vi "GenerateLAB Histo.vi"(9 "Lighting":u16(ring)=5 items=["Incandescent/tungsten", "Old direct sunlight at noon", "Old daylight", "ICC profile PCS", "Mid-morning daylight", "Daylight, sRGB, Adobe-RGB", "North sky daylight", "Equal energy", "Daylight Fluorescent", "Cool fluorescent", "White Fluorescent", "Warm White Fluorescent", "Daylight Fluorescent", "Lite White Fluorescent", "Daylight fluorescent, D65 simulator", "Sylvania F40, D50 simulator", "Cool White Fluorescent", "Ultralume 50, Philips TL85", "Ultralume 40, Philips TL84", "Ultralume 30, Philips TL83"], 11 "2D Picture":picture) -> (1 "Dimensions":string, 3 "Plots":T1)   [LabVIEW 2020]
panel:
  out "b":dbl[](graph)
  out "a":dbl[](graph)
  out "L":dbl[](graph)
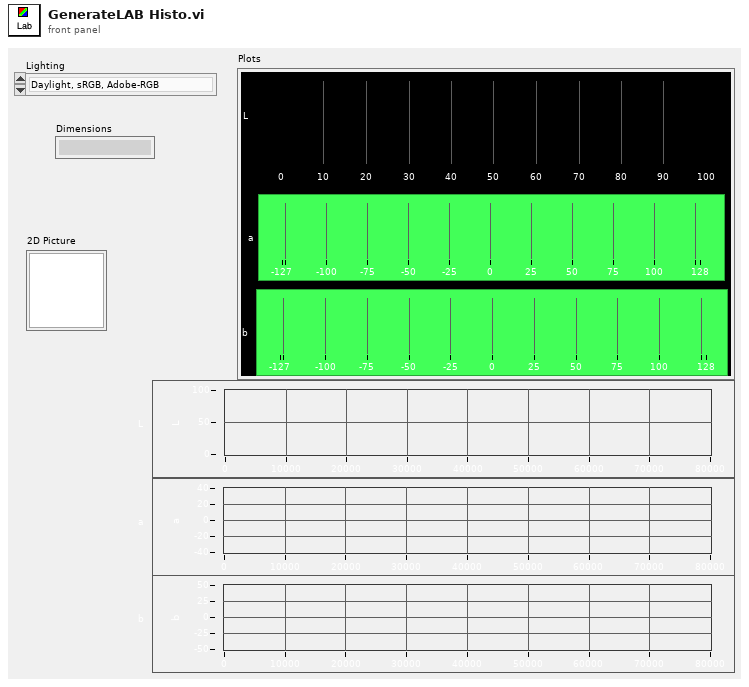
[diagram p1: front panel]
types:
  T1 = cluster{"L":dbl[], "a":cluster{i32, i32, dbl[]}, "b":cluster{i32, i32, dbl[]}}
  T2 = typedef "imagedata.ctl" = cluster{"image type":i32, "image depth":i32, "image":u8[], "mask":u8[], "colors":u32[], "Rectangle":cluster{"left":i16, "top":i16, "right":i16, "bottom":i16}}
  T3 = cluster{dbl[], cluster{i32, i32, dbl[]}, cluster{i32, i32, dbl[]}}
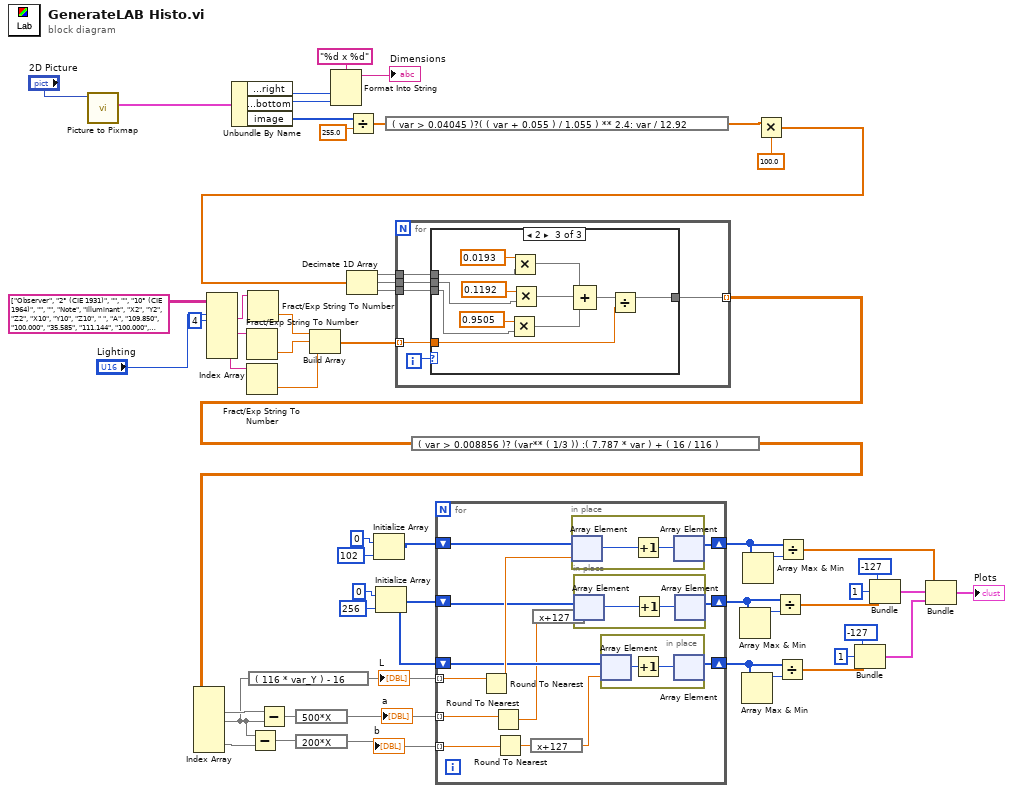
[diagram p0: block diagram]
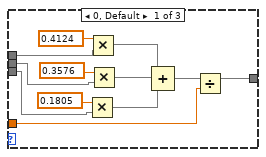
[diagram p2: hidden frame]
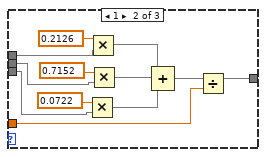
[diagram p3: hidden frame]
diagram:
  n1 = call <vilib>:"Picture to Pixmap.vi"("picture"="2D Picture") -> ("image data"=w1:T2)  [unwired: 9 in, 1 out]
  n2 = Index Array(array=string[][] [["Observer", "2° (CIE 1931)", "", "", "10° (CIE 1964)", "", "", "Note"], ["Illuminant", "X2", "Y2", "Z2", "X10", "Y10", "Z10", " "], ["A", "109.850", "100.000", "35.585", "111.144", "100.000", "35.200", "Incandescent/tungsten"], ["B", "99.0927", "100.000", "85.313", "99.178;", "100.000", "84.3493", "Old direct sunlight at noon"], ["C", "98.074", "100.000", "118.232", "97.285", "100.000", "116.145", "Old daylight"], ["D50", "96.422", "100.000", "82.521", "96.720", "100.000", "81.427", "ICC profile PCS"], ["D55", "95.682", "100.000", "92.149", "95.799", "100.000", "90.926", "Mid-morning daylight"], ["D65", "95.047", "100.000", "108.883", "94.811", "100.000", "107.304", "Daylight, sRGB, Adobe-RGB"], ["D75", "94.972", "100.000", "122.638", "94.416", "100.000", "120.641", "North sky daylight"], ["E", "100.000", "100.000", "100.000", "100.000", "100.000", "100.000", "Equal energy"], ["F1", "92.834", "100.000", "103.665", "94.791", "100.000", "103.191", "Daylight Fluorescent"], ["F2", "99.187", "100.000", "67.395", "103.280", "100.000", "69.026", "Cool fluorescent"], ["F3", "103.754", "100.000", "49.861", "108.968", "100.000", "51.965", "White Fluorescent"], ["F4", "109.147", "100.000", "38.813", "114.961", "100.000", "40.963", "Warm White Fluorescent"], ["F5", "90.872", "100.000", "98.723", "93.369", "100.000", "98.636", "Daylight Fluorescent"], ["F6", "97.309", "100.000", "60.191", "102.148", "100.000", "62.074", "Lite White Fluorescent"], ["F7", "95.044", "100.000", "108.755", "95.792", "100.000", "107.687", "Daylight fluorescent, D65 simulator"], ["F8", "96.413", "100.000", "82.333", "97.115", "100.000", "81.135", "Sylvania F40, D50 simulator"], ["F9", "100.365", "100.000", "67.868", "102.116", "100.000", "67.826", "Cool White Fluorescent"], ["F10", "96.174", "100.000", "81.712", "99.001", "100.000", "83.134", "Ultralume 50, Philips TL85"], ["F11", "100.966", "100.000", "64.370", "103.866", "100.000", "65.627", "Ultralume 40, Philips TL84"], ["F12", "108.046", "100.000", "39.228", "111.428", "100.000", "40.353", "Ultralume 30, Philips TL83"]] ("Table Control"), index (row) #1="Lighting", index (col) #1=4 ("index (col)")) -> (element #1=w14:string, element #2=w13:string, element #3=w12:string)  [unwired: 4 in]
  n3 = Unbundle By Name(w1) -> ("Rectangle.right"=w18:i16, "Rectangle.bottom"=w17:i16, "image"=w39:u8[])
  n4 = Fract/Exp String To Number(string=w13) -> (number=w8:dbl)  [unwired: 3 in, 1 out]
  n5 = Fract/Exp String To Number(string=w12) -> (number=w7:dbl)  [unwired: 3 in, 1 out]
  n6 = Fract/Exp String To Number(string=w14) -> (number=w9:dbl)  [unwired: 3 in, 1 out]
  n7 = Build Array(w9, w8, w7) -> (w6:dbl[])
  n8 = Format Into String(format string="%d x %d", w18, w17) -> (resulting string=→"Dimensions":string)  [unwired: 2 in, 1 out]
  n9 = Divide(x=w39, y=255.0) -> (x/y=w56:dbl[])
  n10 = Initialize Array(u32 0, 102 ("dimension size")) -> (w36:u32[])
  n11 = Initialize Array(u32 0, 256 ("dimension size")) -> (w43:u32[])
  n12 = expression code="( var > 0.04045 )?( ( var + 0.055 ) / 1.055 ) ** 2.4: var / 12.92"(w56) -> (w41:dbl[])
  n13 = Multiply(x=w41, y=100.0) -> (x*y=w40:dbl[])
  n14 = Decimate 1D Array(w40) -> (w55:dbl[], w54:dbl[], w53:dbl[])
  n15 = for {
    tunnel: w55 -> [w62]
    tunnel: w54 -> [w61]
    tunnel: w53 -> [w60]
    tunnel: [w59] -> w52 mode=indexing
    tunnel: w6 -> [w58] mode=indexing
    i -> [w63]
    n16 = case shown="2" w63 {
      tunnel: w62 -> [w74 w86 w98]
      tunnel: w61 -> [w73 w85 w97]
      tunnel: w60 -> [w72 w84 w96]
      tunnel: [w65 w77 w89] -> w59
      tunnel: w58 -> [w64 w76 w88]
      frame 0, Default {
        n17 = Multiply(x=0.1805, y=w72) -> (x*y=w67:dbl[])
        n18 = Multiply(x=0.4124, y=w74) -> (x*y=w68:dbl[])
        n19 = Multiply(x=0.3576, y=w73) -> (x*y=w69:dbl[])
        n20 = Compound Arithmetic op=ADD(w68, w69, w67) -> (w66:dbl[])
        n21 = Divide(x=w66, y=w64) -> (x/y=w65:dbl[])
      }
      frame 1 {
        n22 = Multiply(x=0.0722, y=w84) -> (x*y=w79:dbl[])
        n23 = Multiply(x=0.2126, y=w86) -> (x*y=w80:dbl[])
        n24 = Multiply(x=0.7152, y=w85) -> (x*y=w81:dbl[])
        n25 = Compound Arithmetic op=ADD(w80, w81, w79) -> (w78:dbl[])
        n26 = Divide(x=w78, y=w76) -> (x/y=w77:dbl[])
      }
      frame 2 {
        n27 = Multiply(x=0.9505, y=w96) -> (x*y=w91:dbl[])
        n28 = Multiply(x=0.0193, y=w98) -> (x*y=w92:dbl[])
        n29 = Multiply(x=0.1192, y=w97) -> (x*y=w93:dbl[])
        n30 = Compound Arithmetic op=ADD(w92, w93, w91) -> (w90:dbl[])
        n31 = Divide(x=w90, y=w88) -> (x/y=w89:dbl[])
      }
    }
  }
  n32 = expression code="( var > 0.008856 )? (var** ( 1/3 )) :( 7.787 * var ) + ( 16 / 116 )"(w52) -> (w51:dbl[][])
  n33 = Index Array(array=w51) -> (element #1=w50:dbl[], element #2=w48:dbl[], element #3=w49:dbl[])  [unwired: 6 in]
  n34 = expression code="( 116 * var_Y ) - 16"(w48) -> (w5:dbl[])
  "L" <- w5
  n35 = Subtract(x=w48, y=w49) -> (x-y=w46:dbl[])
  n36 = Subtract(x=w50, y=w48) -> (x-y=w47:dbl[])
  n37 = expression code="500*X"(w47) -> (w3:dbl[])
  "a" <- w3
  n38 = expression code="200*X"(w46) -> (w4:dbl[])
  "b" <- w4
  n39 = for {
    shift-right: [w111] -> w34
    shift-left: w36 -> [w113]
    shift-right: [w108] -> w32
    shift-left: w43 -> [w109]
    shift-right: [w107] -> w30
    shift-left: w43 -> [w110]
    tunnel: w5 -> [w102] mode=indexing
    tunnel: w3 -> [w101] mode=indexing
    tunnel: w4 -> [w100] mode=indexing
    n40 = Round To Nearest(number=w102) -> (nearest integer value=w112:dbl)
    n41 = Round To Nearest(number=w101) -> (nearest integer value=w105:dbl)
    n42 = Round To Nearest(number=w100) -> (nearest integer value=w106:dbl)
    n43 = expression code="x+127"(w106) -> (w103:dbl)
    n44 = expression code="x+127"(w105) -> (w104:dbl)
    n45 = in-place {
      n46 = in-place-array #1(w113, w112) -> (w119:u32)
      n47 = Increment(x=w119) -> (x+1=w118:u32)
      n48 = in-place-array #1(w118) -> (w111:u32[])  [unwired: 1 out]
    }
    n49 = in-place {
      n50 = in-place-array #2(w109, w104) -> (w117:u32)
      n51 = Increment(x=w117) -> (x+1=w116:u32)
      n52 = in-place-array #2(w116) -> (w108:u32[])  [unwired: 1 out]
    }
    n53 = in-place {
      n54 = in-place-array #3(w110, w103) -> (w115:u32)
      n55 = Increment(x=w115) -> (x+1=w114:u32)
      n56 = in-place-array #3(w114) -> (w107:u32[])  [unwired: 1 out]
    }
  }
  n57 = Array Max & Min(array=w32) -> (max value=w33:u32)  [unwired: 3 out]
  n58 = Array Max & Min(array=w30) -> (max value=w31:u32)  [unwired: 3 out]
  n59 = Array Max & Min(array=w34) -> (max value=w35:u32)  [unwired: 3 out]
  n60 = Divide(x=w32, y=w33) -> (x/y=w29:dbl[])
  n61 = Divide(x=w30, y=w31) -> (x/y=w24:dbl[])
  n62 = Divide(x=w34, y=w35) -> (x/y=w23:dbl[])
  n63 = Bundle(-127, 1, w24) -> (w21:cluster{i32, i32, dbl[]})  [unwired: 1 in]
  n64 = Bundle(-127, 1, w29) -> (w22:cluster{i32, i32, dbl[]})  [unwired: 1 in]
  n65 = Bundle(w23, w22, w21) -> (→"Plots":T3)  [unwired: 1 in]
